vi "myRIO_BRig_Host_endExp_storeFiles__v2.vi"(0 "input_filePath":path) -> (6 "output":T1)   [LabVIEW 2014]
panel:
  in  "input_error":errorcluster
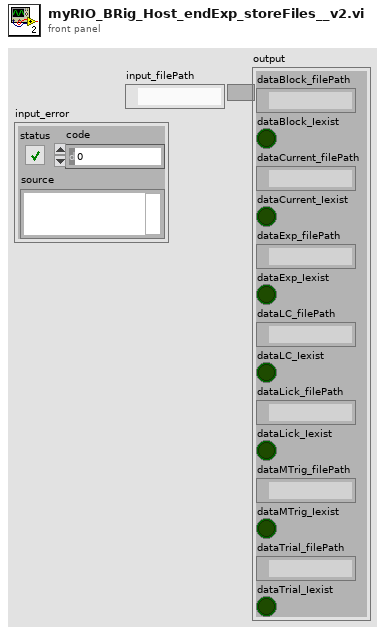
[diagram p1: front panel]
types:
  T1 = cluster{"dataBlock_filePath":path, "dataBlock_Iexist":bool, "dataCurrent_filePath":path, "dataCurrent_Iexist":bool, "dataExp_filePath":path, "dataExp_Iexist":bool, "dataLC_filePath":path, "dataLC_Iexist":bool, "dataLick_filePath":path, "dataLick_Iexist":bool, "dataMTrig_filePath":path, "dataMTrig_Iexist":bool, "dataTrial_filePath":path, "dataTrial_Iexist":bool}
  T2 = cluster{"output_filePath":path, "output_Iexist":bool, "output_filePath":path, "output_Iexist":bool, "output_filePath":path, "output_Iexist":bool, "output_filePath":path, "output_Iexist":bool, "output_filePath":path, "output_Iexist":bool, "output_filePath":path, "output_Iexist":bool, "output_filePath":path, "output_Iexist":bool}
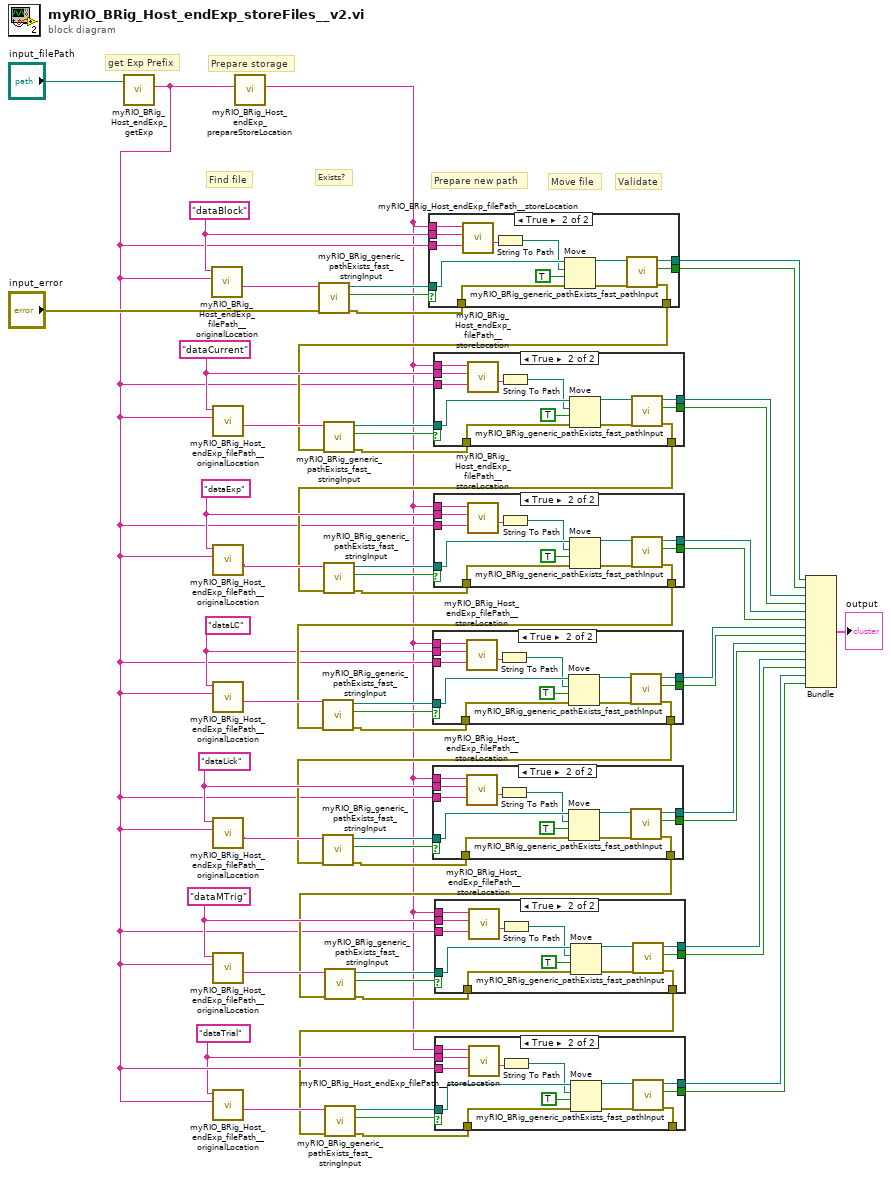
[diagram p0: block diagram]
diagram:
  w18 = "dataTrial" ("input_fileName")
  w25 = "dataMTrig" ("input_fileName")
  w31 = "dataLick" ("input_fileName")
  w36 = "dataLC" ("input_fileName")
  w44 = "dataExp" ("input_fileName")
  w49 = "dataCurrent" ("input_fileName")
  w59 = "dataBlock" ("input_fileName")
  # "Validate"
  # "Move file"
  # "Prepare new path"
  # "Exists?"
  # "Find file"
  # "Prepare storage"
  # "get Exp Prefix"
  n1 = call "myRIO_BRig_Host_endExp_getExp.vi"("input_filePath"="input_filePath") -> ("output_expPrefix"=w19:string)  [unwired: 10 in]
  n2 = call "myRIO_BRig_Host_endExp_filePath__originalLocation.vi"("input_expPrefix"=w19, "input_fileName"=w59) -> ("output_filePath"=w58:string)  [unwired: 9 in]
  n3 = call "myRIO_BRig_Host_endExp_filePath__originalLocation.vi"("input_expPrefix"=w19, "input_fileName"=w49) -> ("output_filePath"=w50:string)  [unwired: 9 in]
  n4 = call "myRIO_BRig_Host_endExp_filePath__originalLocation.vi"("input_expPrefix"=w19, "input_fileName"=w44) -> ("output_filePath"=w45:string)  [unwired: 9 in]
  n5 = call "myRIO_BRig_Host_endExp_filePath__originalLocation.vi"("input_expPrefix"=w19, "input_fileName"=w36) -> ("output_filePath"=w38:string)  [unwired: 9 in]
  n6 = call "myRIO_BRig_Host_endExp_filePath__originalLocation.vi"("input_expPrefix"=w19, "input_fileName"=w31) -> ("output_filePath"=w32:string)  [unwired: 9 in]
  n7 = call "myRIO_BRig_Host_endExp_filePath__originalLocation.vi"("input_expPrefix"=w19, "input_fileName"=w25) -> ("output_filePath"=w26:string)  [unwired: 9 in]
  n8 = call "myRIO_BRig_Host_endExp_filePath__originalLocation.vi"("input_expPrefix"=w19, "input_fileName"=w18) -> ("output_filePath"=w20:string)  [unwired: 9 in]
  n9 = call "myRIO_BRig_Host_endExp_prepareStoreLocation.vi"("input_expPrefix"=w19) -> ("output_folderPath"=w16:string)  [unwired: 9 in, 1 out]
  n10 = call "myRIO_BRig_generic_pathExists_fast_stringInput.vi"("input_error"="input_error", "input_filePath"=w58) -> ("output_error"=w55:errorcluster, "output_Iexist"=w56:bool, "output_filePath"=w57:path)  [unwired: 7 in]
  n11 = case shown="True" w56 {
    selector: w56 -> [w62 _]
    tunnel: w59 -> [_ w75]
    tunnel: w19 -> [_ w76]
    tunnel: w57 -> [w63 w71]
    tunnel: w16 -> [_ w74]
    tunnel: w55 -> [w61 w64]
    tunnel: [w61 w67] -> w43
    tunnel: [w62 w66] -> w14
    tunnel: [w63 w65] -> w15
    frame False {
    }
    frame True {
      n12 = call "myRIO_BRig_Host_endExp_filePath__storeLocation.vi"("input_expPrefix"=w76, "input_fileName"=w75, "input_filePath_storage"=w74) -> ("output_filePath"=w73:string)  [unwired: 8 in]
      n13 = String To Path(string=w73) -> (path=w70:path)
      n14 = Move(source path=w71, error in=w64, 9:TRUE ("overwrite (F)"), 10:w70) -> (error out=w68:errorcluster, 3:w69:path)  [unwired: 1 in, 1 out]
      n15 = call "myRIO_BRig_generic_pathExists_fast_pathInput.vi"("input_error"=w68, "input_filePath"=w69) -> ("output_error"=w67:errorcluster, "output_Iexist"=w66:bool, "output_filePath"=w65:path)  [unwired: 7 in]
    }
  }
  n16 = call "myRIO_BRig_generic_pathExists_fast_stringInput.vi"("input_error"=w43, "input_filePath"=w50) -> ("output_error"=w51:errorcluster, "output_Iexist"=w52:bool, "output_filePath"=w53:path)  [unwired: 7 in]
  n17 = case shown="True" w52 {
    selector: w52 -> [w78 _]
    tunnel: w49 -> [_ w91]
    tunnel: w19 -> [_ w92]
    tunnel: w53 -> [w79 w87]
    tunnel: w16 -> [_ w90]
    tunnel: w51 -> [w77 w80]
    tunnel: [w77 w83] -> w42
    tunnel: [w78 w82] -> w12
    tunnel: [w79 w81] -> w13
    frame False {
    }
    frame True {
      n18 = call "myRIO_BRig_Host_endExp_filePath__storeLocation.vi"("input_expPrefix"=w92, "input_fileName"=w91, "input_filePath_storage"=w90) -> ("output_filePath"=w89:string)  [unwired: 8 in]
      n19 = String To Path(string=w89) -> (path=w86:path)
      n20 = Move(source path=w87, error in=w80, 9:TRUE ("overwrite (F)"), 10:w86) -> (error out=w84:errorcluster, 3:w85:path)  [unwired: 1 in, 1 out]
      n21 = call "myRIO_BRig_generic_pathExists_fast_pathInput.vi"("input_error"=w84, "input_filePath"=w85) -> ("output_error"=w83:errorcluster, "output_Iexist"=w82:bool, "output_filePath"=w81:path)  [unwired: 7 in]
    }
  }
  n22 = call "myRIO_BRig_generic_pathExists_fast_stringInput.vi"("input_error"=w42, "input_filePath"=w45) -> ("output_error"=w46:errorcluster, "output_Iexist"=w47:bool, "output_filePath"=w48:path)  [unwired: 7 in]
  n23 = case shown="True" w47 {
    selector: w47 -> [w94 _]
    tunnel: w44 -> [_ w107]
    tunnel: w19 -> [_ w108]
    tunnel: w48 -> [w95 w103]
    tunnel: w16 -> [_ w106]
    tunnel: w46 -> [w93 w96]
    tunnel: [w93 w99] -> w37
    tunnel: [w94 w98] -> w10
    tunnel: [w95 w97] -> w11
    frame False {
    }
    frame True {
      n24 = call "myRIO_BRig_Host_endExp_filePath__storeLocation.vi"("input_expPrefix"=w108, "input_fileName"=w107, "input_filePath_storage"=w106) -> ("output_filePath"=w105:string)  [unwired: 8 in]
      n25 = String To Path(string=w105) -> (path=w102:path)
      n26 = Move(source path=w103, error in=w96, 9:TRUE ("overwrite (F)"), 10:w102) -> (error out=w100:errorcluster, 3:w101:path)  [unwired: 1 in, 1 out]
      n27 = call "myRIO_BRig_generic_pathExists_fast_pathInput.vi"("input_error"=w100, "input_filePath"=w101) -> ("output_error"=w99:errorcluster, "output_Iexist"=w98:bool, "output_filePath"=w97:path)  [unwired: 7 in]
    }
  }
  n28 = call "myRIO_BRig_generic_pathExists_fast_stringInput.vi"("input_error"=w37, "input_filePath"=w38) -> ("output_error"=w39:errorcluster, "output_Iexist"=w40:bool, "output_filePath"=w41:path)  [unwired: 7 in]
  n29 = case shown="True" w40 {
    selector: w40 -> [w110 _]
    tunnel: w36 -> [_ w123]
    tunnel: w19 -> [_ w124]
    tunnel: w41 -> [w111 w119]
    tunnel: w16 -> [_ w122]
    tunnel: w39 -> [w109 w112]
    tunnel: [w109 w115] -> w30
    tunnel: [w110 w114] -> w8
    tunnel: [w111 w113] -> w9
    frame False {
    }
    frame True {
      n30 = call "myRIO_BRig_Host_endExp_filePath__storeLocation.vi"("input_expPrefix"=w124, "input_fileName"=w123, "input_filePath_storage"=w122) -> ("output_filePath"=w121:string)  [unwired: 8 in]
      n31 = String To Path(string=w121) -> (path=w118:path)
      n32 = Move(source path=w119, error in=w112, 9:TRUE ("overwrite (F)"), 10:w118) -> (error out=w116:errorcluster, 3:w117:path)  [unwired: 1 in, 1 out]
      n33 = call "myRIO_BRig_generic_pathExists_fast_pathInput.vi"("input_error"=w116, "input_filePath"=w117) -> ("output_error"=w115:errorcluster, "output_Iexist"=w114:bool, "output_filePath"=w113:path)  [unwired: 7 in]
    }
  }
  n34 = call "myRIO_BRig_generic_pathExists_fast_stringInput.vi"("input_error"=w30, "input_filePath"=w32) -> ("output_error"=w33:errorcluster, "output_Iexist"=w34:bool, "output_filePath"=w35:path)  [unwired: 7 in]
  n35 = case shown="True" w34 {
    selector: w34 -> [w126 _]
    tunnel: w31 -> [_ w139]
    tunnel: w19 -> [_ w140]
    tunnel: w35 -> [w127 w135]
    tunnel: w16 -> [_ w138]
    tunnel: w33 -> [w125 w128]
    tunnel: [w125 w131] -> w24
    tunnel: [w126 w130] -> w2
    tunnel: [w127 w129] -> w7
    frame False {
    }
    frame True {
      n36 = call "myRIO_BRig_Host_endExp_filePath__storeLocation.vi"("input_expPrefix"=w140, "input_fileName"=w139, "input_filePath_storage"=w138) -> ("output_filePath"=w137:string)  [unwired: 8 in]
      n37 = String To Path(string=w137) -> (path=w134:path)
      n38 = Move(source path=w135, error in=w128, 9:TRUE ("overwrite (F)"), 10:w134) -> (error out=w132:errorcluster, 3:w133:path)  [unwired: 1 in, 1 out]
      n39 = call "myRIO_BRig_generic_pathExists_fast_pathInput.vi"("input_error"=w132, "input_filePath"=w133) -> ("output_error"=w131:errorcluster, "output_Iexist"=w130:bool, "output_filePath"=w129:path)  [unwired: 7 in]
    }
  }
  n40 = call "myRIO_BRig_generic_pathExists_fast_stringInput.vi"("input_error"=w24, "input_filePath"=w26) -> ("output_error"=w27:errorcluster, "output_Iexist"=w28:bool, "output_filePath"=w29:path)  [unwired: 7 in]
  n41 = case shown="True" w28 {
    selector: w28 -> [w142 _]
    tunnel: w25 -> [_ w155]
    tunnel: w19 -> [_ w156]
    tunnel: w29 -> [w143 w151]
    tunnel: w16 -> [_ w154]
    tunnel: w27 -> [w141 w144]
    tunnel: [w141 w147] -> w17
    tunnel: [w142 w146] -> w3
    tunnel: [w143 w145] -> w6
    frame False {
    }
    frame True {
      n42 = call "myRIO_BRig_Host_endExp_filePath__storeLocation.vi"("input_expPrefix"=w156, "input_fileName"=w155, "input_filePath_storage"=w154) -> ("output_filePath"=w153:string)  [unwired: 8 in]
      n43 = String To Path(string=w153) -> (path=w150:path)
      n44 = Move(source path=w151, error in=w144, 9:TRUE ("overwrite (F)"), 10:w150) -> (error out=w148:errorcluster, 3:w149:path)  [unwired: 1 in, 1 out]
      n45 = call "myRIO_BRig_generic_pathExists_fast_pathInput.vi"("input_error"=w148, "input_filePath"=w149) -> ("output_error"=w147:errorcluster, "output_Iexist"=w146:bool, "output_filePath"=w145:path)  [unwired: 7 in]
    }
  }
  n46 = call "myRIO_BRig_generic_pathExists_fast_stringInput.vi"("input_error"=w17, "input_filePath"=w20) -> ("output_error"=w21:errorcluster, "output_Iexist"=w22:bool, "output_filePath"=w23:path)  [unwired: 7 in]
  n47 = case shown="True" w22 {
    selector: w22 -> [w158 _]
    tunnel: w18 -> [_ w171]
    tunnel: w19 -> [_ w172]
    tunnel: w23 -> [w159 w167]
    tunnel: w16 -> [_ w170]
    tunnel: w21 -> [w157 w160]
    tunnel: [w157 w163] -> _
    tunnel: [w158 w162] -> w4
    tunnel: [w159 w161] -> w5
    frame False {
    }
    frame True {
      n48 = call "myRIO_BRig_Host_endExp_filePath__storeLocation.vi"("input_expPrefix"=w172, "input_fileName"=w171, "input_filePath_storage"=w170) -> ("output_filePath"=w169:string)  [unwired: 8 in]
      n49 = String To Path(string=w169) -> (path=w166:path)
      n50 = Move(source path=w167, error in=w160, 9:TRUE ("overwrite (F)"), 10:w166) -> (error out=w164:errorcluster, 3:w165:path)  [unwired: 1 in, 1 out]
      n51 = call "myRIO_BRig_generic_pathExists_fast_pathInput.vi"("input_error"=w164, "input_filePath"=w165) -> ("output_error"=w163:errorcluster, "output_Iexist"=w162:bool, "output_filePath"=w161:path)  [unwired: 7 in]
    }
  }
  n52 = Bundle("output_filePath"=w15, "output_Iexist"=w14, "output_filePath"=w13, "output_Iexist"=w12, "output_filePath"=w11, "output_Iexist"=w10, "output_filePath"=w9, "output_Iexist"=w8, "output_filePath"=w7, "output_Iexist"=w2, "output_filePath"=w6, "output_Iexist"=w3, "output_filePath"=w5, "output_Iexist"=w4) -> (→"output":T2)  [unwired: 1 in]
